vi "Scale Vector.vi"(8 "error in":errorcluster, 10 "n (1)":dbl=1.0, 11 "PVector V":refnum<class "PVector.lvclass">) -> (0 "error out":errorcluster, 3 "PVector nV":refnum<class "PVector.lvclass">)   [LabVIEW 2016, in "PVector.lvclass"]
doc: "Scale vector V by scalar <B>n</B>.\nScales each of the vector components : \nnV == n(Vx,Vy) == (nVx,nVy)"
uses:
  PVector.lvclass
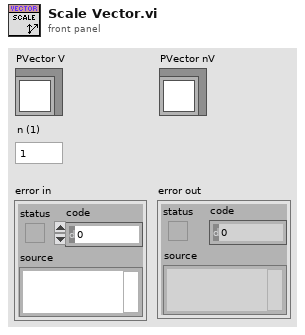
[diagram p1: front panel]
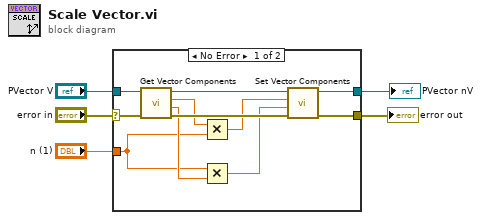
[diagram p0: block diagram]
diagram:
  n1 = case shown="No Error" "error in" {
    selector: "error in" -> [w15 w18]
    tunnel: [w8 w18] -> w4
    tunnel: [w13 w17] -> w2
    tunnel: "PVector V" -> [w16 w17]
    tunnel: "n (1)" -> [w9 _]
    frame No Error {
      n2 = call "Get Vector Components.vi"("error in"=w15, "PVector in"=w16) -> ("error out"=w12:errorcluster, "Y"=w10:dbl, "X"=w11:dbl, "PVector out"=w14:refnum<class "PVector.lvclass">)  [unwired: 6 in]
      n3 = Multiply(x=w11, y=w9) -> (x*y=w7:dbl)
      n4 = Multiply(x=w9, y=w10) -> (x*y=w6:dbl)
      n5 = call "Set Vector Components.vi"("error in"=w12, "Y"=w6, "X"=w7, "PVector in"=w14) -> ("error out"=w8:errorcluster, "PVector out"=w13:refnum<class "PVector.lvclass">)  [unwired: 6 in]
    }
    frame Error {
    }
  }
  "error out" <- w4
  "PVector nV" <- w2
